vi "RNN-Node.vi"(0 "Weight_Length":i32, 1 "Wight_Start_Index":i16, 2 "Bias":i16, 3 "Input_Array":i16[](array[numeric]), 4 "Weight_Array":i16[](array[numeric])) -> (5 "Output":i16)   [LabVIEW 2020]
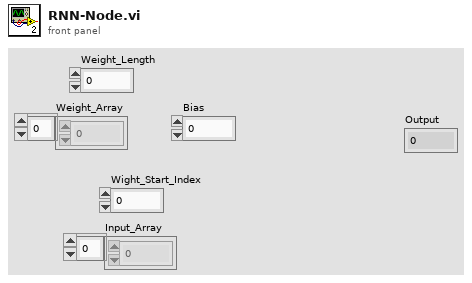
[diagram p1: front panel]
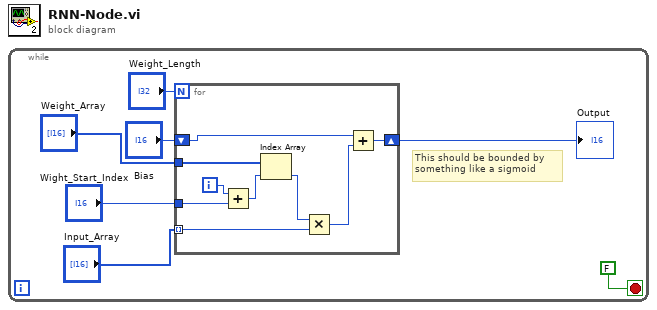
[diagram p0: block diagram]
diagram:
  n1 = while {
    stop <- FALSE stop-if-true
    # "This should be bounded by \nsomething like a sigmoid"
    n2 = for {
      N: "Weight_Length" -> [_]
      tunnel: "Weight_Array" -> [w16]
      shift-right: [w14] -> w3
      shift-left: "Bias" -> [w15]
      tunnel: "Wight_Start_Index" -> [w12]
      tunnel: "Input_Array" -> [w9] mode=indexing
      i -> [w11]
      n3 = Add(x=w11, y=w12) -> (x+y=w13:i32)
      n4 = Index Array(array=w16, index=w13) -> (element=w10:i16)
      n5 = Multiply(x=w10, y=w9) -> (x*y=w8:i16)
      n6 = Add(x=w15, y=w8) -> (x+y=w14:i16)
    }
    "Output" <- w3
  }
